vi "Set Report Tab Width.vi"(0 "report in":refnum<class "NI_Standard Report.lvclass">, 5 "width (.25)":dbl=0.25 format="%.2f", 9 "measurement system (US)":u16(ring) items=["US", "Metric"], 11 "error in (no error)":errorcluster) -> (4 "report out":refnum<class "NI_Standard Report.lvclass">, 15 "error out":errorcluster)   [LabVIEW 2015, in "NI_Standard Report.lvclass"]
doc: "Sets the tab width in the report. You cannot use this VI with HTML, Word, and Excel reports."
uses:
  <vilib>/Utility/NIReport.llb/Standard Report/NI_Standard Report.lvclass
  <vilib>/Utility/NIReport.llb/Standard Report/NI_Standard Report.lvclass/NI_Standard Report.ctl
  <vilib>/Utility/NIReport.llb/NI_ReportGenerationCore.lvlib
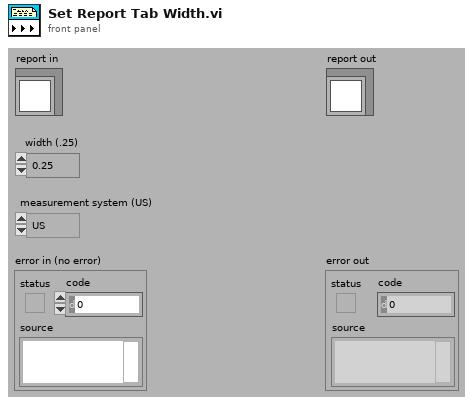
[diagram p1: front panel]
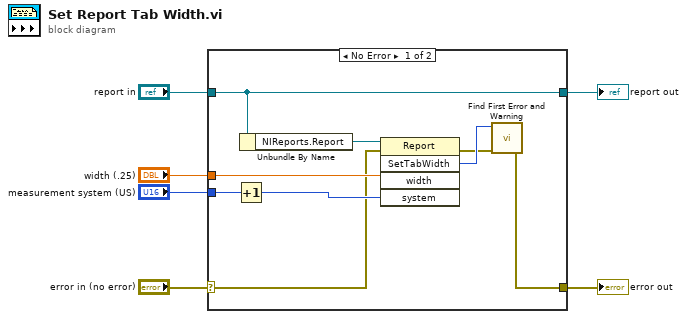
[diagram p0: block diagram]
diagram:
  n1 = case shown="No Error" "error in (no error)" {
    selector: "error in (no error)" -> [w8 w17]
    tunnel: [w7 w17] -> w5
    tunnel: [w11 w16] -> w3
    tunnel: "report in" -> [w11 w16]
    tunnel: "width (.25)" -> [w10 _]
    tunnel: "measurement system (US)" -> [w9 _]
    frame No Error {
      n2 = Increment(x=w9) -> (x+1=w15:u16)
      n3 = Unbundle By Name(w11) -> ("NIReports.Report"=w12:refnum<k7>)
      n4 = invoke class="Report" method="SetTabWidth"(reference=w12, error in=w8, "width"=w10, "system"=w15) -> (error out=w13:errorcluster, "SetTabWidth"=w14:i32)  [unwired: 1 in, 3 out]
      n5 = call <vilib>:"Find First Error and Warning.vi"("error in (no error)"=w13, "error code"=w14) -> ("error out"=w7:errorcluster)  [unwired: 1 in, 4 out]
    }
    frame Error {
    }
  }
  "error out" <- w5
  "report out" <- w3
